vi "PE7260_Volt_conv.vi"(0 "Numerisch":dbl) -> (1 "Numerisch 2":dbl, 2 "String":string)   [LabVIEW 2018]
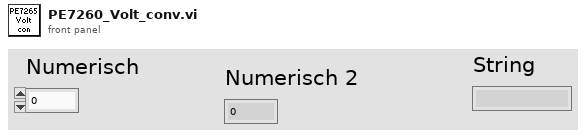
[diagram p1: front panel]
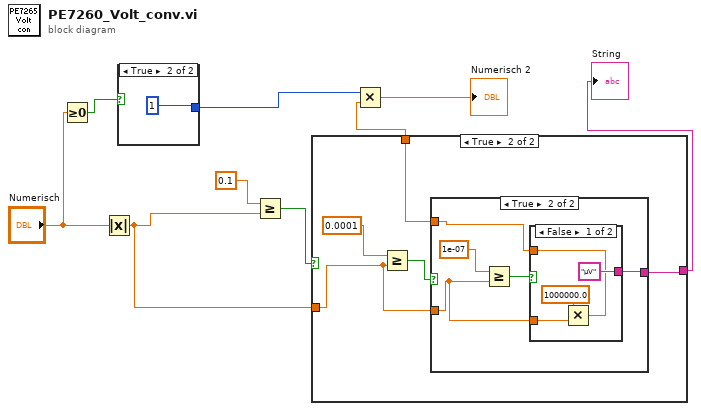
[diagram p0: block diagram]
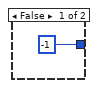
[diagram p2: hidden frame]
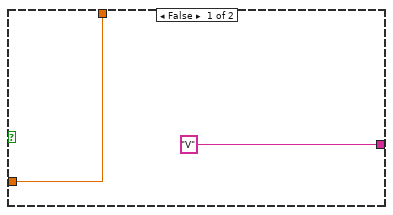
[diagram p3: hidden frame]
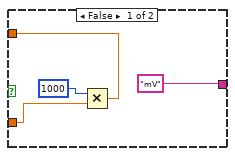
[diagram p4: hidden frame]
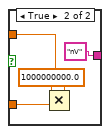
[diagram p5: hidden frame]
diagram:
  n1 = Greater Or Equal To 0?(x="Numerisch") -> (x >= 0?=w4:bool)
  n2 = Absolute Value(x="Numerisch") -> (abs(x)=w6:dbl)
  n3 = case shown="True" w4 {
    tunnel: [-1 1] -> w1
    frame False {
    }
    frame True {
    }
  }
  n4 = Greater Or Equal?(x=0.1, y=w6) -> (x >= y?=w8:bool)
  n5 = case shown="True" w8 {
    tunnel: w6 -> [w12 w15]
    tunnel: ["V" w16] -> w7
    tunnel: [w12 w14] -> w3
    frame False {
    }
    frame True {
      n6 = Greater Or Equal?(x=0.0001, y=w15) -> (x >= y?=w17:bool)
      n7 = case shown="True" w17 {
        tunnel: ["mV" w27] -> w16
        tunnel: w15 -> [w20 w24]
        tunnel: [w19 w23] -> w14
        frame False {
          n8 = Multiply(x=1000, y=w20) -> (x*y=w19:dbl)
        }
        frame True {
          n9 = Greater Or Equal?(x=1e-07, y=w24) -> (x >= y?=w26:bool)
          n10 = case shown="False" w26 {
            tunnel: ["µV" "nV"] -> w27
            tunnel: w24 -> [w30 w35]
            tunnel: [w28 w33] -> w23
            frame False {
              n11 = Multiply(x=1000000.0, y=w30) -> (x*y=w28:dbl)
            }
            frame True {
              n12 = Multiply(x=1000000000.0, y=w35) -> (x*y=w33:dbl)
            }
          }
        }
      }
    }
  }
  "String" <- w7
  n13 = Multiply(x=w1, y=w3) -> (x*y=→"Numerisch 2":dbl)
